vi "ABCtoAlphaBeta_2PhaseUnitaryMagnitude_src.vi"(0 "A":sgl, 5 "B":sgl) -> (4 "alpha":sgl, 6 "beta":sgl)   [LabVIEW 2015]
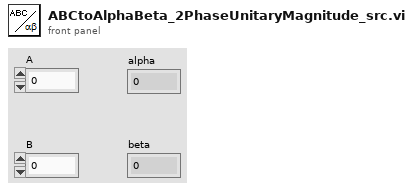
[diagram p1: front panel]
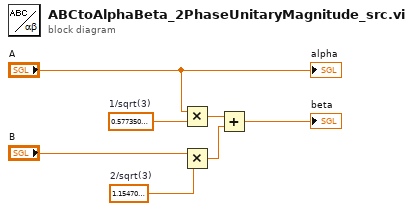
[diagram p0: block diagram]
diagram:
  w1 = sgl 1.1547005  # 2/sqrt(3)
  w2 = sgl 0.57735026  # 1/sqrt(3)
  n1 = Multiply(x="A", y=w2) -> (x*y=w7:sgl)
  n2 = Multiply(x="B", y=w1) -> (x*y=w6:sgl)
  n3 = Add(x=w7, y=w6) -> (x+y=→"beta":sgl)
  "alpha" <- "A"
